vi "Write.vi"(0 "Arduino Resource in":T2, 5 "Register":T1, 9 "Value":u8, 11 "error in (no error)":errorcluster) -> (4 "Arduino Resource Out":T2, 15 "error out":errorcluster)   [LabVIEW 2012, in "Digital Compass HMC5883L.lvlib"]
doc: "Only the first three registers are writable (Config A, Config B, Mode)"
uses:
  Digital Compass HMC5883L.lvlib
  <vilib>/LabVIEW Interface for Arduino/Type Defs/Arduino Resource.ctl
  <vilib>/LabVIEW Interface for Arduino/Type Defs/Board Type.ctl
  Registers.ctl
  <vilib>/LabVIEW Interface for Arduino/LabVIEW Interface for Arduino.lvlib
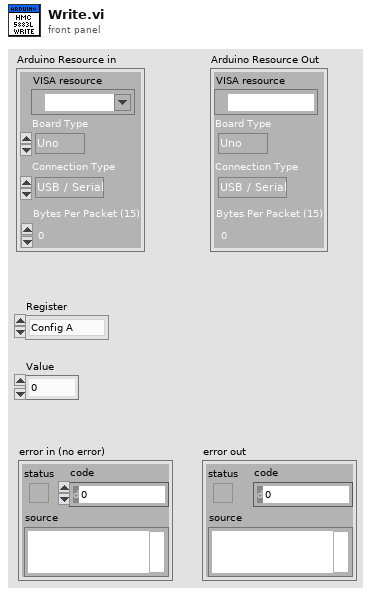
[diagram p1: front panel]
types:
  T1 = typedef "Digital Compass HMC5883L.lvlib/Registers.ctl" = enum16{"Config A", "Config B", "Mode", "X MSB", "X LSB", "Z MSB", "Z LSB", "Y MSB", "Y LSB", "Status", "ID A", "ID B", "ID C"}
  T2 = typedef "LabVIEW Interface for Arduino.lvlib/Arduino Resource.ctl" = cluster{"VISA resource":refnum<visa-resource-name>, "Board Type":T3, "Connection Type":enum8{"USB / Serial"}, "Bytes Per Packet (15)":u8}
  T3 = typedef "LabVIEW Interface for Arduino.lvlib/Board Type.ctl" = enum16{"Uno", "Dimuelanove w/Atmega 328", "Mega 2560"}
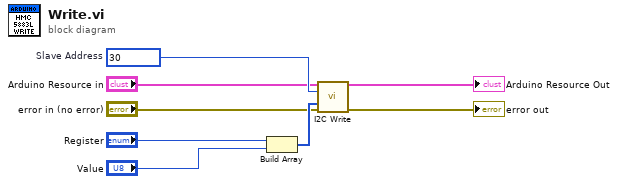
[diagram p0: block diagram]
diagram:
  w8 = u8 30  # Slave Address
  n1 = Build Array("Register", "Value") -> (w7:u16[])
  n2 = call <vilib>:"I2C Write.vi"("Arduino Resource"="Arduino Resource in", "Address (0)"=w8, "I2C Data Bytes"=w7, "error in"="error in (no error)") -> ("Arduino Resource"=→"Arduino Resource Out":T2, "error out"=→"error out":errorcluster)  [unwired: 10 in]
